vi "Check for Data.vi"(4 "error in (no error)":errorcluster, 7 "Statement Refnum":T1) -> (0 "error out":errorcluster, 2 "Data Present?":bool, 3 "Statement Refnum":T1)   [LabVIEW 2011]
doc: "Charge la prochaine ligne et établit si elle est vide. Dans ce cas, ferme le curseur de la requête"
uses:
  SQL Controls/Statement Refnum.ctl
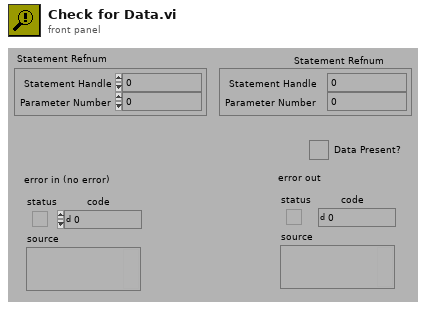
[diagram p1: front panel]
types:
  T1 = typedef "Statement Refnum.ctl" = cluster{"Statement Handle":i32, "Parameter Number":u16}
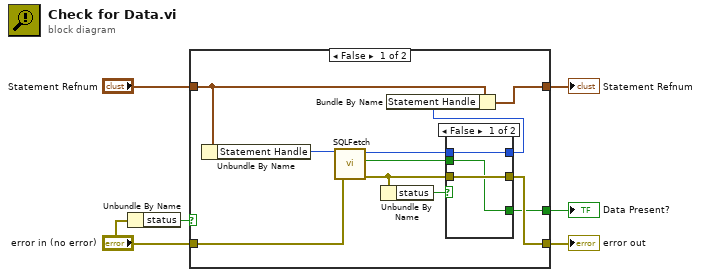
[diagram p0: block diagram]
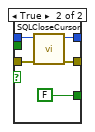
[diagram p2: hidden frame]
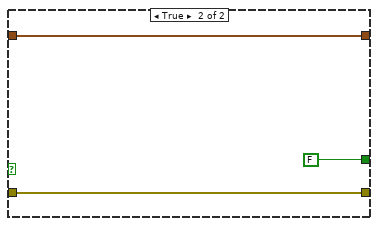
[diagram p3: hidden frame]
diagram:
  n1 = Unbundle By Name("error in (no error)") -> ("status"=w3:bool)
  n2 = case shown="False" w3 {
    tunnel: "Statement Refnum" -> [w17 w28]
    tunnel: [w7 FALSE] -> w1
    tunnel: [w15 w28] -> w5
    tunnel: [w10 w27] -> w2
    tunnel: "error in (no error)" -> [w12 w27]
    frame False {
      n3 = Unbundle By Name(w17) -> ("Statement Handle"=w13:i32)
      n4 = call "SQLFetch.vi"("error in (no error)"=w12, "InputHandle"=w13) -> ("error out"=w11:errorcluster, "Data Present?"=w8:bool, "OutputHandle"=w14:i32)  [unwired: 1 in, 2 out]
      n5 = Unbundle By Name(w11) -> ("status"=w9:bool)
      n6 = case shown="False" w9 {
        tunnel: [w20 w25] -> w16
        tunnel: w14 -> [w20 w24]
        tunnel: w11 -> [w19 w23]
        tunnel: [w19 w22] -> w10
        tunnel: [w18 FALSE] -> w7
        tunnel: w8 -> [w18 _]
        frame False {
        }
        frame True {
          n7 = call "SQLCloseCursor.vi"("error in (no error)"=w23, "InputHandle"=w24) -> ("error out"=w22:errorcluster, "OutputHandle"=w25:i32)  [unwired: 4 out]
        }
      }
      n8 = Bundle By Name(cluster=w17, "Statement Handle"=w16) -> (w15:T1)
    }
    frame True {
    }
  }
  "Data Present?" <- w1
  "Statement Refnum" <- w5
  "error out" <- w2
